vi "MD5 Message Digest (Hexadecimal String)__ogtk.vi"(1 "Message":string) -> (0 "MD5 Message Digest":string)   [LabVIEW 2016]
doc: "Implements the MD5 algorithm to produce a 128-Bit Hash condensed representation of a message or a data file.\n\nPolymorphic VI can output MD5 Hash as Binary String or Hexadeximal String."
panel:
  # "Please visit http://www.OpenG.org to learn about the\nOpen Source LabVIEW software movement.\n\nNOTICE -- YOU MUST LEAVE THIS NOTICE IN PLACE.  PER THE TERMS OF THE LICENSE BELOW, YOU MAY SUBLICENSE THIS SOFTWARE \nIN ANY WAY THAT DOES NOT CONFLICT WITH THIS LICENSE.\n\n### BSD License (http://www.opensource.org/licenses/bsd-license.php) Begin ###\n \nCopyright (c) 2004, Enrique Vargas <vargas@visecurity.com>\nCopyright (c) 2011, Jonathon Green <jg@jgcode.net>\n\nAll rights reserved.\n\nRedistribution and use in source and binary forms, with or without modification, are permitted provided that the following conditions are met:\n\n    * Redistributions of source code must retain the above copyright notice, this list of conditions and the following disclaimer.\n    * Redistributions in binary form must reproduce the above copyright notice, this list of conditions and the following disclaimer in the \n       documentation and/or other materials provided with the distribution.\n    * Neither the name of SciWare, James Kring, Inc., nor the names of its contributors may be used to endorse or promote products derived \n       from this software without specific prior written permission.\n\nTHIS SOFTWARE IS PROVIDED BY THE COPYRIGHT HOLDERS AND CONTRIBUTORS \"AS IS\" AND ANY EXPRESS OR IMPLIED WARRANTIES, \nINCLUDING, BUT NOT LIMITED TO, THE IMPLIED WARRANTIES OF MERCHANTABILITY AND FITNESS FOR A PARTICULAR PURPOSE ARE \nDISCLAIMED. IN NO EVENT SHALL THE COPYRIGHT OWNER OR CONTRIBUTORS BE LIABLE FOR ANY DIRECT, INDIRECT, INCIDENTAL,\n SPECIAL, EXEMPLARY, OR CONSEQUENTIAL DAMAGES (INCLUDING, BUT NOT LIMITED TO, PROCUREMENT OF SUBSTITUTE GOODS OR \nSERVICES; LOSS OF USE, DATA, OR PROFITS; OR BUSINESS INTERRUPTION) HOWEVER CAUSED AND ON ANY THEORY OF LIABILITY, \nWHETHER IN CONTRACT, STRICT LIABILITY, OR TORT (INCLUDING NEGLIGENCE OR OTHERWISE) ARISING IN ANY WAY OUT OF THE USE \nOF THIS SOFTWARE, EVEN IF ADVISED OF THE POSSIBILITY OF SUCH DAMAGE.\n\n### BSD License End ###"
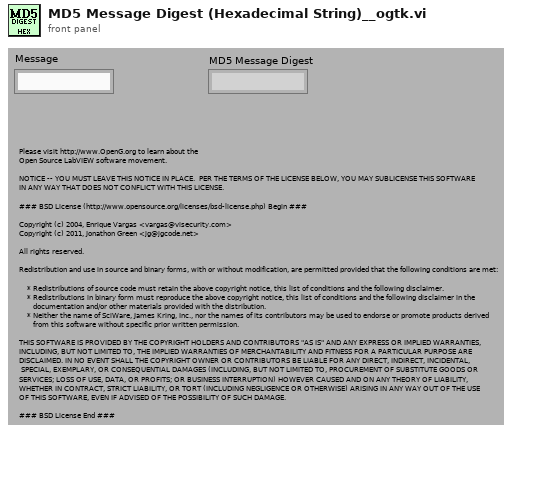
[diagram p1: front panel]
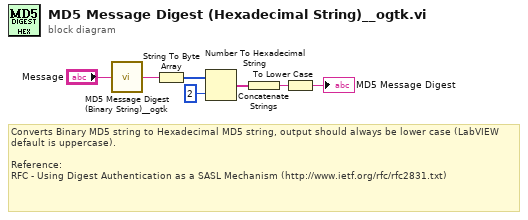
[diagram p0: block diagram]
diagram:
  # "Converts Binary MD5 string to Hexadecimal MD5 string, output should always be lower case (LabVIEW default is uppercase).\n\nReference:\nRFC - Using Digest Authentication as a SASL Mechanism (http://www.ietf.org/rfc/rfc2831.txt)"
  n1 = call "MD5 Message Digest (Binary String)__ogtk.vi"("Message"="Message") -> ("MD5 Message Digest"=w3:string)
  n2 = String To Byte Array(string=w3) -> (unsigned byte array=w6:u8[])
  n3 = Number To Hexadecimal String(1:i16 2 ("width (-)"), 2:w6) -> (0:w5:string[])
  n4 = Concatenate Strings(w5) -> (w4:string)
  n5 = To Lower Case(string=w4) -> (all lower case string=→"MD5 Message Digest":string)
